vi "ToString.vi"(8 "error in (no error)":errorcluster, 11 "String Ends With in":refnum<class "String Ends With.lvclass">) -> (0 "error out":errorcluster, 2 "String":string, 3 "String Ends With out":refnum<class "String Ends With.lvclass">)   [LabVIEW 2017, in "Transparent Assertions.lvlib" / "String Ends With.lvclass"]
doc: "Returns a string representation of the object."
uses:
  String Ends With.lvclass
  String Ends With.lvclass/String Ends With.ctl
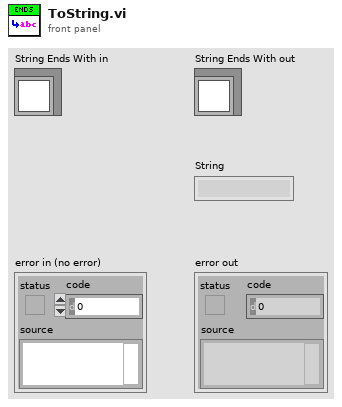
[diagram p1: front panel]
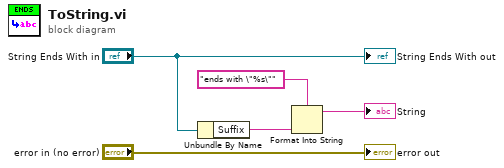
[diagram p0: block diagram]
diagram:
  n1 = Unbundle By Name("String Ends With in") -> ("Suffix"=w1:string)
  n2 = Format Into String(format string="ends with \"%s\"", w1) -> (resulting string=→"String":string)  [unwired: 2 in, 1 out]
  "error out" <- "error in (no error)"
  "String Ends With out" <- "String Ends With in"
